vi "PosCentersBackAreaQuadrada.vi"(8 "Robô fora?":bool=TRUE, 9 "geometry":T1, 10 "Defensores":u32[](array[numeric]), 11 "Pos Bola":dbl[](array[numeric]) format="%#_13g") -> (2 "Pos Centers Back":dbl[][](array[numeric]), 3 "Central Position":dbl[](array[numeric]))   [LabVIEW 2017]
uses:
  Core/Field Size.ctl
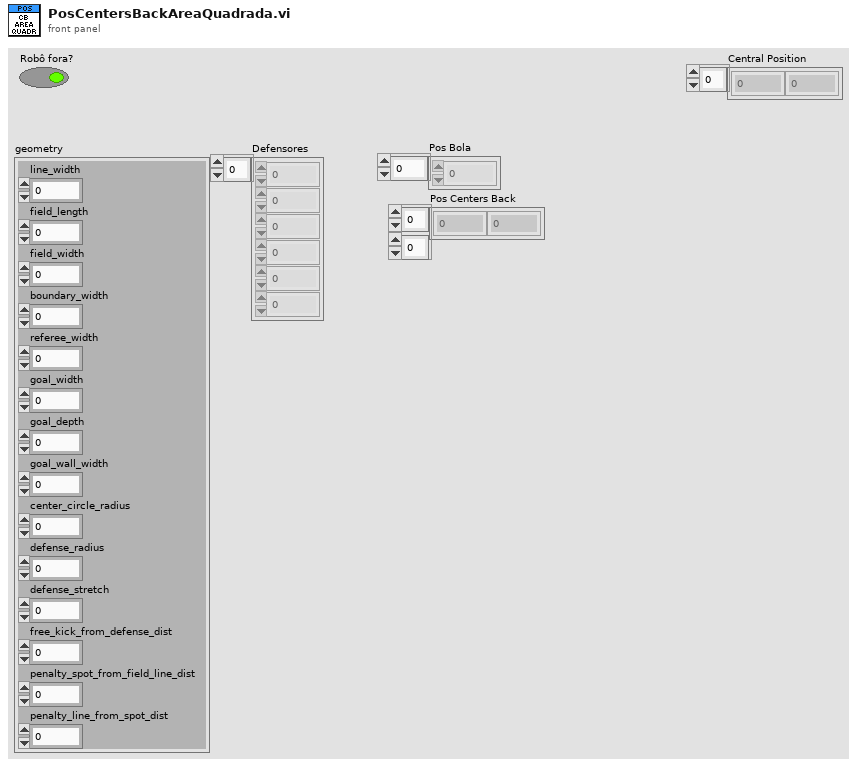
[diagram p1: front panel]
types:
  T1 = typedef "Field Size.ctl" = cluster{"line_width":u32, "field_length":u32, "field_width":u32, "boundary_width":u32, "referee_width":u32, "goal_width":u32, "goal_depth":u32, "goal_wall_width":u32, "center_circle_radius":u32, "defense_radius":u32, "defense_stretch":u32, "free_kick_from_defense_dist":u32, "penalty_spot_from_field_line_dist":u32, "penalty_line_from_spot_dist":u32}
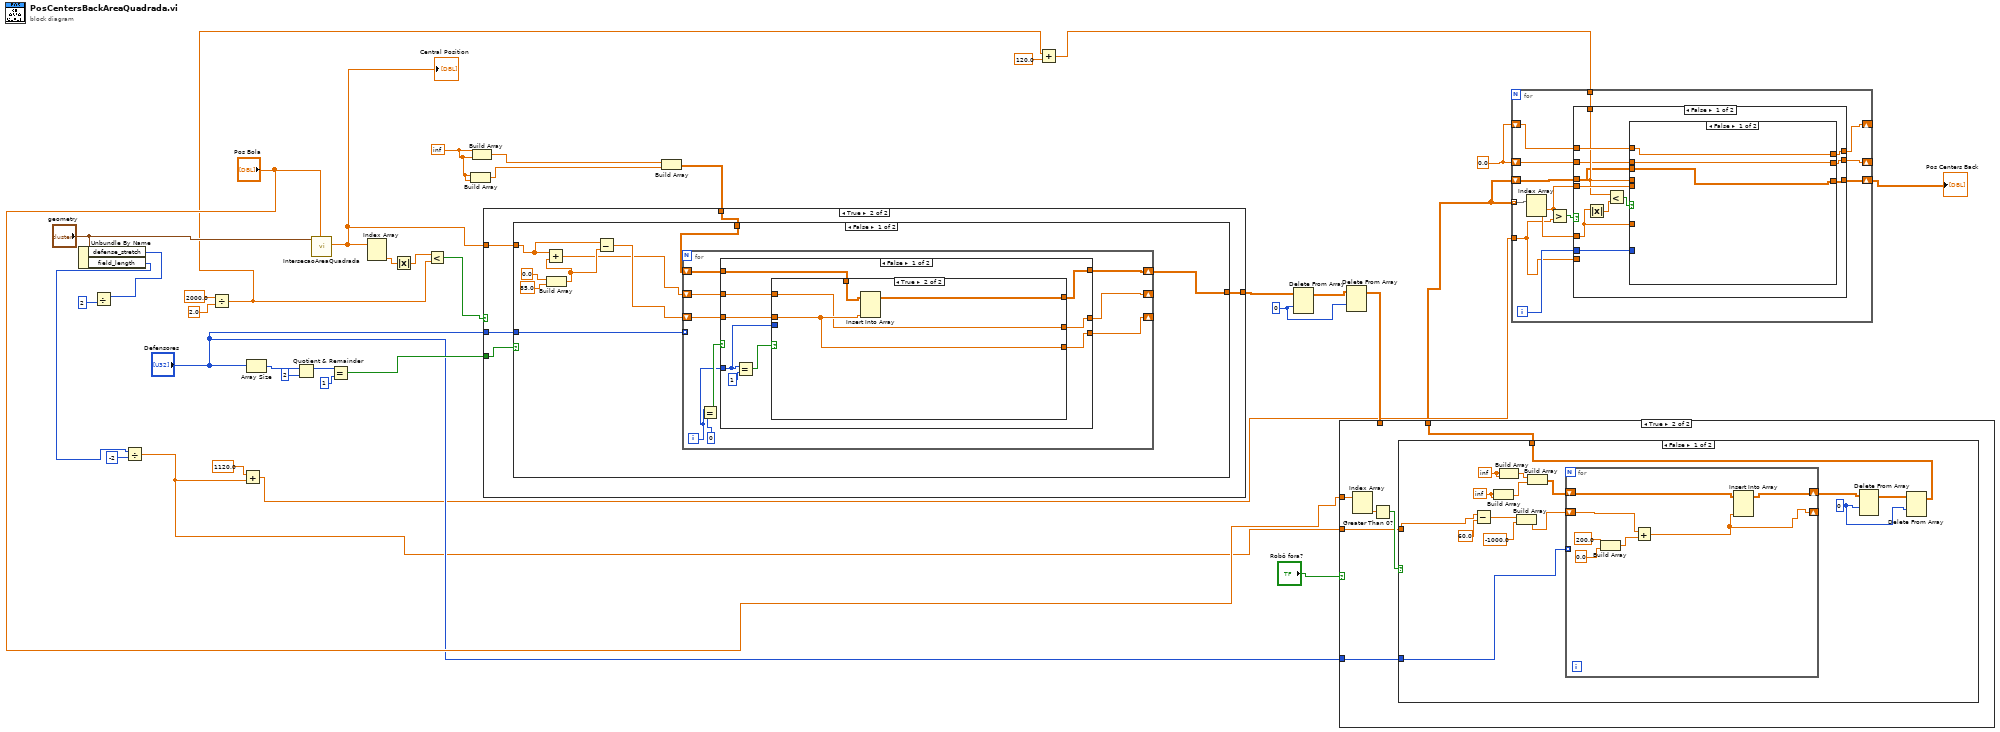
[diagram p0: block diagram]
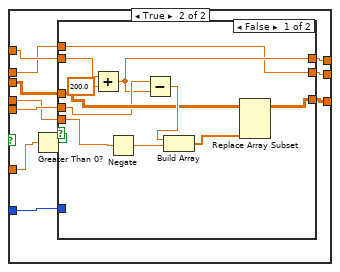
[diagram p2: hidden frame]
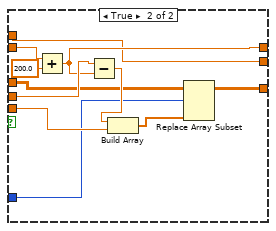
[diagram p3: hidden frame]
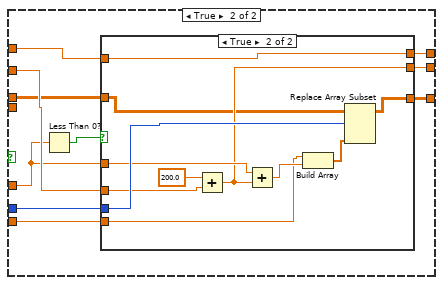
[diagram p4: hidden frame]
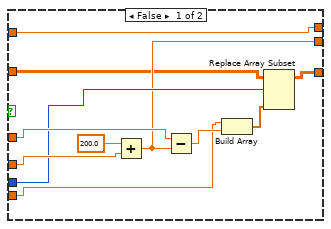
[diagram p5: hidden frame]
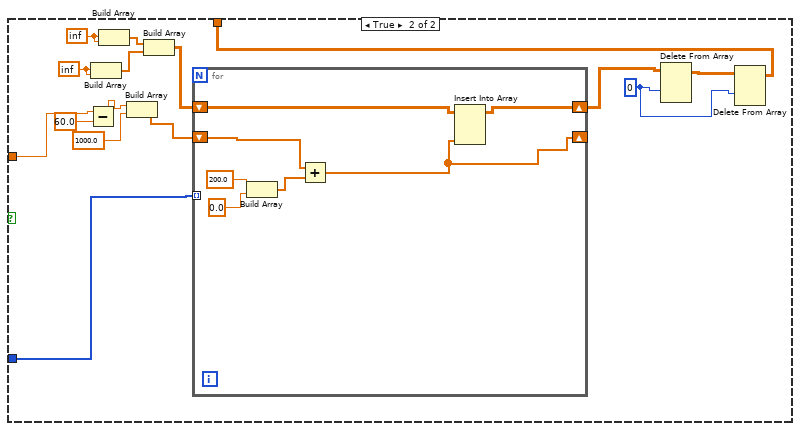
[diagram p7: hidden frame]
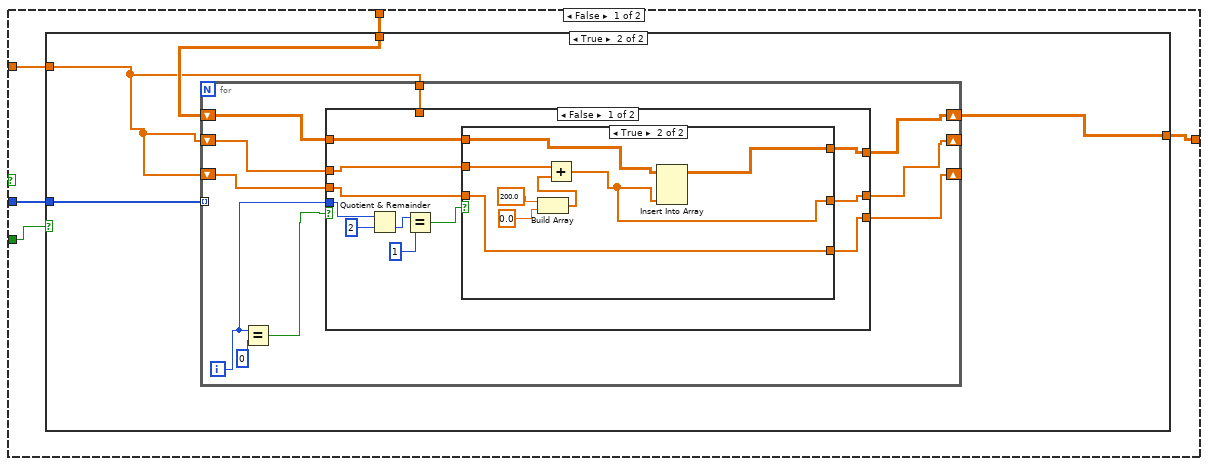
[diagram p8: hidden frame]
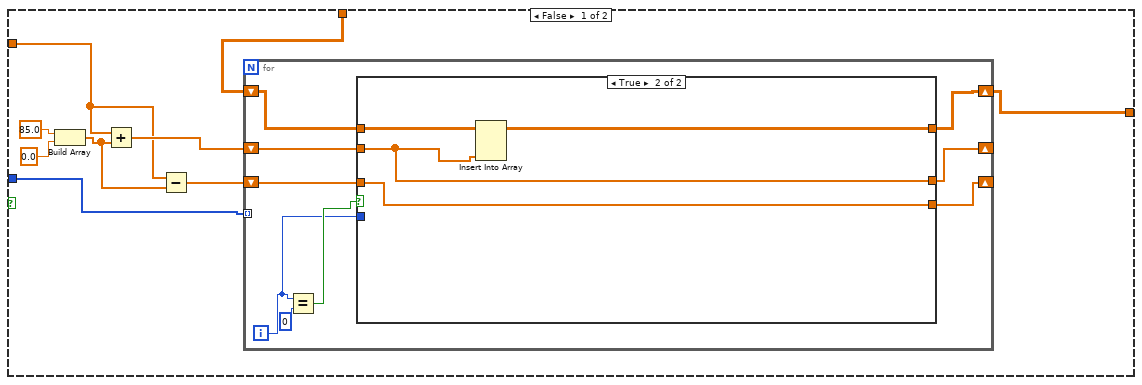
[diagram p9: hidden frame]
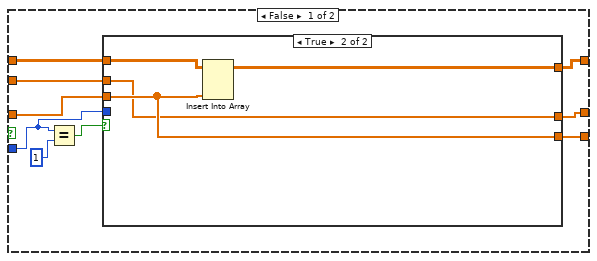
[diagram p10: hidden frame]
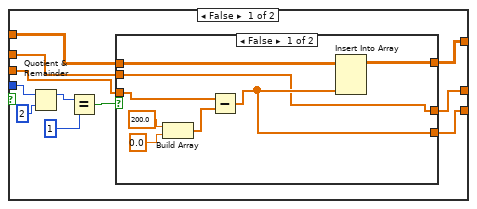
[diagram p11: hidden frame]
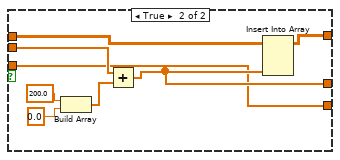
[diagram p12: hidden frame]
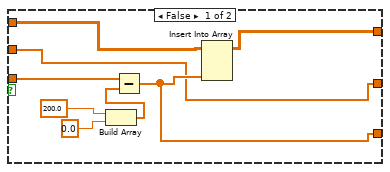
[diagram p13: hidden frame]
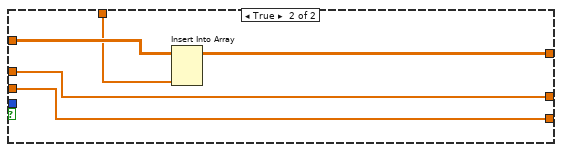
[diagram p14: hidden frame]
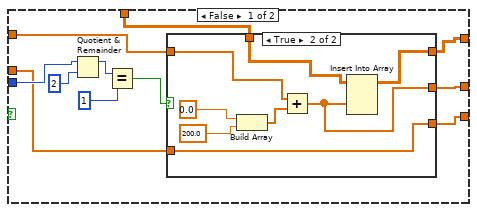
[diagram p15: hidden frame]
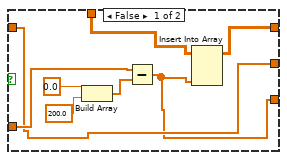
[diagram p16: hidden frame]
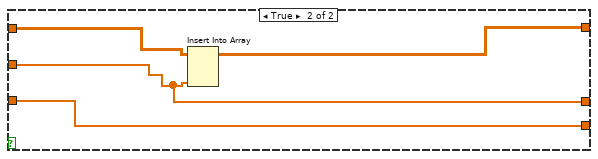
[diagram p17: hidden frame]
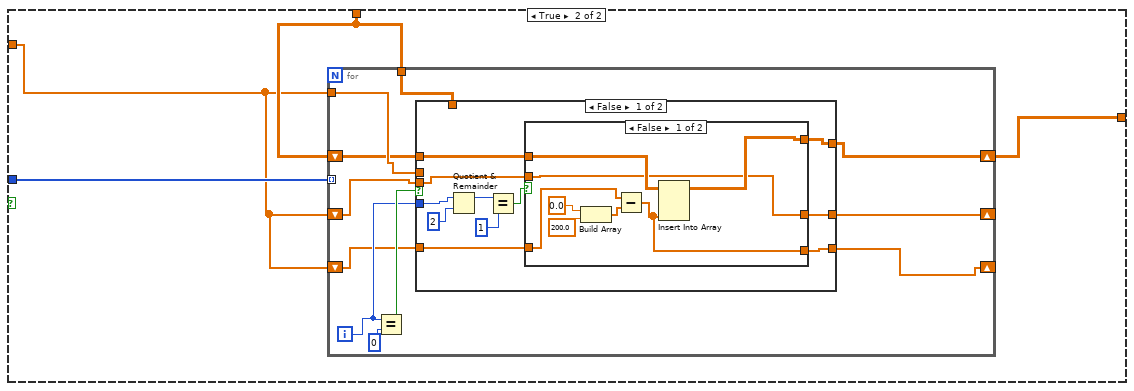
[diagram p18: hidden frame]
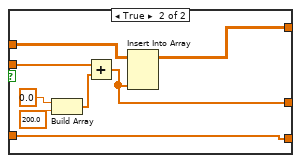
[diagram p19: hidden frame]
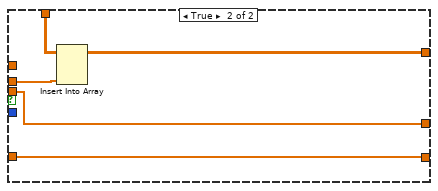
[diagram p20: hidden frame]
diagram:
  w5 = 0.0
  w17 = 0 ("index (row)")
  w23 = inf
  n1 = Unbundle By Name("geometry") -> ("defense_stretch"=w35:u32, "field_length"=w12:u32)
  n2 = Divide(x=w35, y=u32 2) -> ()  [unwired: 1 out]
  n3 = Divide(x=w12, y=-2) -> (x/y=w6:dbl)
  n4 = Divide(x=2000.0, y=2.0) -> (x/y=w2:dbl)
  n5 = Add(x=1120.0 ("y"), y=w6) -> (x+y=w9:dbl)
  n6 = Array Size(array="Defensores") -> (size(s)=w28:i32)
  n7 = Quotient & Remainder(x=w28, y=2) -> (x-y*floor(x/y)=w26:i32)  [unwired: 1 out]
  n8 = call "IntersecaoAreaQuadrada.vi"("Pos entrada"="Pos Bola", "geometry"="geometry") -> ("Pos de Interseção"=w16:dbl[])  [unwired: 8 in, 1 out]
  "Central Position" <- w16
  n9 = Equal?(x=w26, y=1) -> (x = y?=w24:bool)
  n10 = Index Array(array=w16) -> (element #2=w31:dbl)  [unwired: 2 in, 1 out]
  n11 = Absolute Value(x=w31) -> (abs(x)=w30:dbl)
  n12 = Less?(x=w30, y=w2) -> (x < y?=w29:bool)
  n13 = Build Array(w23, w23) -> (w21:dbl[])
  n14 = Build Array(w23, w23) -> (w22:dbl[])
  n15 = Build Array(w22, w21) -> (w20:dbl[][])
  n16 = case shown="True" w29 {
    tunnel: w24 -> [w41 w154]
    tunnel: "Defensores" -> [w40 w153]
    tunnel: w16 -> [w38 w152]
    tunnel: w20 -> [w39 w151]
    tunnel: [w37 w150] -> w19
    frame False {
      n17 = case shown="True" w41 {
        tunnel: w40 -> [w42 w107]
        tunnel: w39 -> [w44 w106]
        tunnel: w38 -> [w47 w105]
        tunnel: [w43 w104] -> w37
        frame False {
          n18 = Build Array(85.0, 0.0) -> (w46:dbl[])
          n19 = Add(x=w47, y=w46) -> (x+y=w48:dbl[])
          n20 = Subtract(x=w47, y=w46) -> (x-y=w45:dbl[])
          n21 = for {
            shift-right: [w54] -> _
            shift-left: w48 -> [w56]
            shift-right: [w53] -> _
            shift-left: w45 -> [w52]
            shift-right: [w55] -> w43
            shift-left: w44 -> [w57]
            tunnel: w42 -> [_] mode=indexing
            i -> [w51]
            n22 = Equal?(x=w51, y=0) -> (x = y?=w58:bool)
            n23 = case shown="True" w58 {
              tunnel: w57 -> [w66 w103]
              tunnel: w56 -> [w62 w101]
              tunnel: [w61 w102] -> w55
              tunnel: [w63 w101] -> w54
              tunnel: [w64 w100] -> w53
              tunnel: w52 -> [w65 w100]
              tunnel: w51 -> [w60 _]
              frame False {
                n24 = Equal?(x=w60, y=1) -> (x = y?=w67:bool)
                n25 = case shown="True" w67 {
                  tunnel: w66 -> [w74 w99]
                  tunnel: w65 -> [w69 w98]
                  tunnel: [w70 w98] -> w64
                  tunnel: [w71 w97] -> w63
                  tunnel: w62 -> [w73 w97]
                  tunnel: [w72 w96] -> w61
                  tunnel: w60 -> [w79 _]
                  frame False {
                    n26 = Quotient & Remainder(x=w79, y=2) -> (x-y*floor(x/y)=w77:i32)  [unwired: 1 out]
                    n27 = Equal?(x=w77, y=1) -> (x = y?=w75:bool)
                    n28 = case shown="False" w75 {
                      tunnel: w74 -> [w86 w95]
                      tunnel: w73 -> [w80 w91]
                      tunnel: [w87 w90] -> w72
                      tunnel: [w80 w89] -> w71
                      tunnel: [w81 w88] -> w70
                      tunnel: w69 -> [w82 w88]
                      frame False {
                        n29 = Build Array(200.0, 0.0) -> (w83:dbl[])
                        n30 = Subtract(x=w82, y=w83) -> (x-y=w81:dbl[])
                        n31 = Insert Into Array(array=w86, new element=w81) -> (w87:dbl[][])  [unwired: 2 in]
                      }
                      frame True {
                        n32 = Build Array(200.0, 0.0) -> (w92:dbl[])
                        n33 = Add(x=w91, y=w92) -> (x+y=w89:dbl[])
                        n34 = Insert Into Array(array=w95, new element=w89) -> (w90:dbl[][])  [unwired: 2 in]
                      }
                    }
                  }
                  frame True {
                    n35 = Insert Into Array(array=w99, new element=w98) -> (w96:dbl[][])  [unwired: 2 in]
                  }
                }
              }
              frame True {
                n36 = Insert Into Array(array=w103, new element=w101) -> (w102:dbl[][])  [unwired: 2 in]
              }
            }
          }
        }
        frame True {
          n37 = for {
            tunnel: w107 -> [_] mode=indexing
            shift-right: [w113] -> w104
            shift-left: w106 -> [w115]
            shift-right: [w111] -> _
            shift-left: w105 -> [w110]
            shift-right: [w109] -> _
            shift-left: w105 -> [w108]
            tunnel: w105 -> [w114]
            i -> [w112]
            n38 = Equal?(x=w112, y=0) -> (x = y?=w116:bool)
            n39 = case shown="False" w116 {
              tunnel: w115 -> [w123 w149]
              tunnel: w114 -> [_ w148]
              tunnel: [w122 w147] -> w113
              tunnel: w112 -> [w128 _]
              tunnel: [w119 w146] -> w111
              tunnel: w110 -> [w124 w146]
              tunnel: [w120 w145] -> w109
              tunnel: w108 -> [w121 w145]
              frame False {
                n40 = Quotient & Remainder(x=w128, y=2) -> (floor(x/y)=w126:i32)  [unwired: 1 out]
                n41 = Equal?(x=w126, y=1) -> (x = y?=w118:bool)
                n42 = case shown="True" w118 {
                  tunnel: w124 -> [w130 w142]
                  tunnel: w123 -> [w133 w140]
                  tunnel: [w132 w139] -> w122
                  tunnel: w121 -> [w134 w138]
                  tunnel: [w131 w138] -> w120
                  tunnel: [w130 w137] -> w119
                  frame False {
                    n43 = Build Array(200.0, 0.0 ("element")) -> (w135:dbl[])
                    n44 = Subtract(x=w134, y=w135) -> (x-y=w131:dbl[])
                    n45 = Insert Into Array(array=w133, new element=w131) -> (w132:dbl[][])  [unwired: 2 in]
                  }
                  frame True {
                    n46 = Build Array(200.0, 0.0) -> (w141:dbl[])
                    n47 = Add(x=w142, y=w141) -> (x+y=w137:dbl[])
                    n48 = Insert Into Array(array=w140, new element=w137) -> (w139:dbl[][])  [unwired: 2 in]
                  }
                }
              }
              frame True {
                n49 = Insert Into Array(array=w149, new element=w148) -> (w147:dbl[][])  [unwired: 2 in]
              }
            }
          }
        }
      }
    }
    frame True {
      n50 = case shown="False" w154 {
        tunnel: w153 -> [w163 w220]
        tunnel: w152 -> [w160 w218]
        tunnel: w151 -> [w158 w219]
        tunnel: [w155 w217] -> w150
        frame False {
          n51 = Build Array(0.0, 85.0) -> (w159:dbl[])
          n52 = Add(x=w160, y=w159) -> (x+y=w156:dbl[])
          n53 = Subtract(x=w160, y=w159) -> (x-y=w157:dbl[])
          n54 = for {
            tunnel: w163 -> [_] mode=indexing
            shift-right: [w164] -> _
            shift-left: w156 -> [w169]
            shift-right: [w168] -> w155
            shift-left: w158 -> [w170]
            shift-right: [w165] -> _
            shift-left: w157 -> [w166]
            i -> [w167]
            n55 = Equal?(x=w167, y=0) -> (x = y?=w171:bool)
            n56 = case shown="False" w171 {
              tunnel: w170 -> [w179 w216]
              tunnel: w169 -> [w174 w213]
              tunnel: [w177 w215] -> w168
              tunnel: w167 -> [w173 _]
              tunnel: w166 -> [w178 w214]
              tunnel: [w176 w214] -> w165
              tunnel: [w175 w213] -> w164
              frame False {
                n57 = Equal?(x=w173, y=1) -> (x = y?=w180:bool)
                n58 = case shown="True" w180 {
                  tunnel: w179 -> [w187 w212]
                  tunnel: w178 -> [w183 w210]
                  tunnel: [w186 w211] -> w177
                  tunnel: [w184 w210] -> w176
                  tunnel: [w185 w209] -> w175
                  tunnel: w174 -> [w188 w209]
                  tunnel: w173 -> [w192 _]
                  frame False {
                    n59 = Quotient & Remainder(x=w192, y=2) -> (x-y*floor(x/y)=w182:i32)  [unwired: 1 out]
                    n60 = Equal?(x=w182, y=1) -> (x = y?=w189:bool)
                    n61 = case shown="True" w189 {
                      tunnel: w188 -> [w194 w205]
                      tunnel: w187 -> [w195 w204]
                      tunnel: [w196 w203] -> w186
                      tunnel: [w194 w202] -> w185
                      tunnel: [w193 w201] -> w184
                      tunnel: w183 -> [w197 w201]
                      frame False {
                        n62 = Build Array(0.0, 200.0) -> (w200:dbl[])
                        n63 = Subtract(x=w197, y=w200) -> (x-y=w193:dbl[])
                        n64 = Insert Into Array(array=w195, new element=w193) -> (w196:dbl[][])  [unwired: 2 in]
                      }
                      frame True {
                        n65 = Build Array(0.0, 200.0) -> (w206:dbl[])
                        n66 = Add(x=w205, y=w206) -> (x+y=w202:dbl[])
                        n67 = Insert Into Array(array=w204, new element=w202) -> (w203:dbl[][])  [unwired: 2 in]
                      }
                    }
                  }
                  frame True {
                    n68 = Insert Into Array(array=w212, new element=w210) -> (w211:dbl[][])  [unwired: 2 in]
                  }
                }
              }
              frame True {
                n69 = Insert Into Array(array=w216, new element=w213) -> (w215:dbl[][])  [unwired: 2 in]
              }
            }
          }
        }
        frame True {
          n70 = for {
            tunnel: w220 -> [_] mode=indexing
            tunnel: w219 -> [w230]
            tunnel: w218 -> [w229]
            shift-right: [w228] -> w217
            shift-left: w219 -> [w225]
            shift-right: [w223] -> _
            shift-left: w218 -> [w224]
            shift-right: [w221] -> _
            shift-left: w218 -> [w222]
            i -> [w226]
            n71 = Equal?(x=w226, y=0) -> (x = y?=w231:bool)
            n72 = case shown="False" w231 {
              tunnel: w230 -> [_ w263]
              tunnel: w229 -> [_ w262]
              tunnel: [w236 w261] -> w228
              tunnel: w226 -> [w242 _]
              tunnel: w225 -> [w237 _]
              tunnel: w224 -> [w235 w260]
              tunnel: [w234 w260] -> w223
              tunnel: w222 -> [w233 w259]
              tunnel: [w232 w259] -> w221
              frame False {
                n73 = Quotient & Remainder(x=w242, y=2) -> (x-y*floor(x/y)=w240:i32)  [unwired: 1 out]
                n74 = Equal?(x=w240, y=1) -> (x = y?=w238:bool)
                n75 = case shown="False" w238 {
                  tunnel: w237 -> [w246 w255]
                  tunnel: [w245 w254] -> w236
                  tunnel: w235 -> [w243 w253]
                  tunnel: [w243 w252] -> w234
                  tunnel: w233 -> [w247 w251]
                  tunnel: [w244 w251] -> w232
                  frame False {
                    n76 = Build Array(0.0, 200.0) -> (w248:dbl[])
                    n77 = Subtract(x=w247, y=w248) -> (x-y=w244:dbl[])
                    n78 = Insert Into Array(array=w246, new element=w244) -> (w245:dbl[][])  [unwired: 2 in]
                  }
                  frame True {
                    n79 = Build Array(0.0, 200.0) -> (w256:dbl[])
                    n80 = Add(x=w253, y=w256) -> (x+y=w252:dbl[])
                    n81 = Insert Into Array(array=w255, new element=w252) -> (w254:dbl[][])  [unwired: 2 in]
                  }
                }
              }
              frame True {
                n82 = Insert Into Array(array=w263, new element=w262) -> (w261:dbl[][])  [unwired: 2 in]
              }
            }
          }
        }
      }
    }
  }
  n83 = Add(x=w2, y=120.0) -> (x+y=w1:dbl)
  n84 = Delete From Array(array=w19, index (row)=w17) -> (array with subset deleted=w18:dbl[][])  [unwired: 2 in, 1 out]
  n85 = Delete From Array(array=w18, index (row)=w17) -> (array with subset deleted=w13:dbl[][])  [unwired: 2 in, 1 out]
  n86 = case shown="True" "Robô fora?" {
    tunnel: "Pos Bola" -> [_ w270]
    tunnel: [w264 w265] -> w8
    tunnel: w13 -> [w264 _]
    tunnel: w6 -> [_ w267]
    tunnel: "Defensores" -> [_ w266]
    frame False {
    }
    frame True {
      n87 = Index Array(array=w270) -> (element #2=w269:dbl)  [unwired: 2 in, 1 out]
      n88 = Greater Than 0?(x=w269) -> (x > 0?=w268:bool)
      n89 = case shown="False" w268 {
        tunnel: w267 -> [w273 w295]
        tunnel: w266 -> [w275 w306]
        tunnel: [w274 w296] -> w265
        frame False {
          w276 = 0 ("index (row)")
          w281 = inf
          w280 = inf
          n90 = Subtract(x=w273, y=60.0) -> (x-y=w271:dbl)
          n91 = Build Array(w281, w281) -> (w283:dbl[])
          n92 = Build Array(w280, w280) -> (w282:dbl[])
          n93 = Build Array(w271, -1000.0) -> (w284:dbl[])
          n94 = Build Array(w282, w283) -> (w279:dbl[][])
          n95 = for {
            tunnel: w275 -> [_] mode=indexing
            shift-right: [w287] -> w278
            shift-left: w279 -> [w288]
            shift-right: [w286] -> _
            shift-left: w284 -> [w289]
            n96 = Build Array(200.0, 0.0) -> (w290:dbl[])
            n97 = Add(x=w289, y=w290) -> (x+y=w286:dbl[])
            n98 = Insert Into Array(array=w288, new element=w286) -> (w287:dbl[][])  [unwired: 2 in]
          }
          n99 = Delete From Array(array=w278, index (row)=w276) -> (array with subset deleted=w277:dbl[][])  [unwired: 2 in, 1 out]
          n100 = Delete From Array(array=w277, index (row)=w276) -> (array with subset deleted=w274:dbl[][])  [unwired: 2 in, 1 out]
        }
        frame True {
          w297 = 0 ("index (row)")
          w302 = inf
          w301 = inf
          n101 = Subtract(x=w295, y=60.0) -> (x-y=w293:dbl)
          n102 = Build Array(w302, w302) -> (w304:dbl[])
          n103 = Build Array(w301, w301) -> (w303:dbl[])
          n104 = Build Array(w293, 1000.0) -> (w305:dbl[])
          n105 = Build Array(w303, w304) -> (w300:dbl[][])
          n106 = for {
            tunnel: w306 -> [_] mode=indexing
            shift-right: [w309] -> w299
            shift-left: w300 -> [w310]
            shift-right: [w308] -> _
            shift-left: w305 -> [w311]
            n107 = Build Array(200.0, 0.0) -> (w312:dbl[])
            n108 = Add(x=w311, y=w312) -> (x+y=w308:dbl[])
            n109 = Insert Into Array(array=w310, new element=w308) -> (w309:dbl[][])  [unwired: 2 in]
          }
          n110 = Delete From Array(array=w299, index (row)=w297) -> (array with subset deleted=w298:dbl[][])  [unwired: 2 in, 1 out]
          n111 = Delete From Array(array=w298, index (row)=w297) -> (array with subset deleted=w296:dbl[][])  [unwired: 2 in, 1 out]
        }
      }
    }
  }
  n112 = for {
    tunnel: w8 -> [w325] mode=indexing
    tunnel: w9 -> [w322]
    shift-right: [w321] -> _
    shift-left: w5 -> [w323]
    shift-right: [w319] -> w4
    shift-left: w8 -> [w320]
    tunnel: w1 -> [w318]
    shift-right: [w315] -> _
    shift-left: w5 -> [w317]
    i -> [w324]
    n113 = Index Array(array=w325) -> (element #1=w316:dbl, element #2=w326:dbl)  [unwired: 2 in]
    n114 = Greater?(x=w316, y=w322) -> (0:w327:bool)
    n115 = case shown="False" w327 {
      tunnel: w326 -> [w337 w382]
      tunnel: w324 -> [w332 w384]
      tunnel: w323 -> [w329 w383]
      tunnel: w322 -> [_ w381]
      tunnel: [w328 w380] -> w321
      tunnel: w320 -> [w331 w379]
      tunnel: [w330 w378] -> w319
      tunnel: w318 -> [w333 _]
      tunnel: w317 -> [w336 w376]
      tunnel: w316 -> [w335 _]
      tunnel: [w334 w377] -> w315
      frame False {
        n116 = Absolute Value(x=w337) -> (abs(x)=w339:dbl)
        n117 = Less?(x=w333, y=w339) -> (x < y?=w338:bool)
        n118 = case shown="False" w338 {
          tunnel: w337 -> [_ w353]
          tunnel: w336 -> [w341 w351]
          tunnel: w335 -> [_ w350]
          tunnel: [w341 w349] -> w334
          tunnel: w333 -> [_ w348]
          tunnel: w332 -> [_ w347]
          tunnel: w331 -> [w342 w346]
          tunnel: [w342 w345] -> w330
          tunnel: w329 -> [w340 w344]
          tunnel: [w340 w343] -> w328
          frame False {
          }
          frame True {
            n119 = Greater Than 0?(x=w353) -> (x > 0?=w352:bool)
            n120 = case shown="False" w352 {
              tunnel: w351 -> [w359 w375]
              tunnel: w350 -> [w358 w373]
              tunnel: [w355 w372] -> w349
              tunnel: w348 -> [w356 w370]
              tunnel: w347 -> [_ w369]
              tunnel: w346 -> [w360 w367]
              tunnel: [w361 w366] -> w345
              tunnel: w344 -> [w354 w365]
              tunnel: [w354 w365] -> w343
              frame False {
                n121 = Add(x=w359, y=200.0) -> (x+y=w355:dbl)
                n122 = Negate(x=w356) -> (-x=w357:dbl)
                n123 = Subtract(x=w358, y=w355) -> (x-y=w363:dbl)
                n124 = Build Array(w363, w357) -> (w362:dbl[])
                n125 = Replace Array Subset(array=w360, new element=w362) -> (w361:dbl[][])  [unwired: 2 in]
              }
              frame True {
                n126 = Add(x=w375, y=200.0) -> (x+y=w372:dbl)
                n127 = Subtract(x=w373, y=w372) -> (x-y=w371:dbl)
                n128 = Build Array(w371, w370) -> (w368:dbl[])
                n129 = Replace Array Subset(array=w367, new element=w368, index (row)=w369) -> (w366:dbl[][])  [unwired: 1 in]
              }
            }
          }
        }
      }
      frame True {
        n130 = Less Than 0?(x=w382) -> (x < 0?=w385:bool)
        n131 = case shown="True" w385 {
          tunnel: w384 -> [w392 w407]
          tunnel: w383 -> [w394 w406]
          tunnel: w382 -> [w393 w404]
          tunnel: w381 -> [w391 w401]
          tunnel: [w390 w400] -> w380
          tunnel: w379 -> [w389 w399]
          tunnel: [w388 w398] -> w378
          tunnel: [w387 w397] -> w377
          tunnel: w376 -> [w387 w397]
          frame False {
            n132 = Add(x=200.0, y=w394) -> (x+y=w390:dbl)
            n133 = Subtract(x=w393, y=w390) -> (x-y=w396:dbl)
            n134 = Build Array(w391, w396) -> (w395:dbl[])
            n135 = Replace Array Subset(array=w389, new element=w395, index (row)=w392) -> (w388:dbl[][])  [unwired: 1 in]
          }
          frame True {
            n136 = Add(x=200.0, y=w406) -> (x+y=w400:dbl)
            n137 = Add(x=w404, y=w400) -> (x+y=w403:dbl)
            n138 = Build Array(w401, w403) -> (w402:dbl[])
            n139 = Replace Array Subset(array=w399, new element=w402, index (row)=w407) -> (w398:dbl[][])  [unwired: 1 in]
          }
        }
      }
    }
  }
  "Pos Centers Back" <- w4
